vi "Sample Array - Fix Ascii.vi"(11 "Sample Array In":string[](array[string])) -> (3 "Sample Array Out":string[](array[string]))   [LabVIEW 2012]
uses:
  Globals Wilt.vi
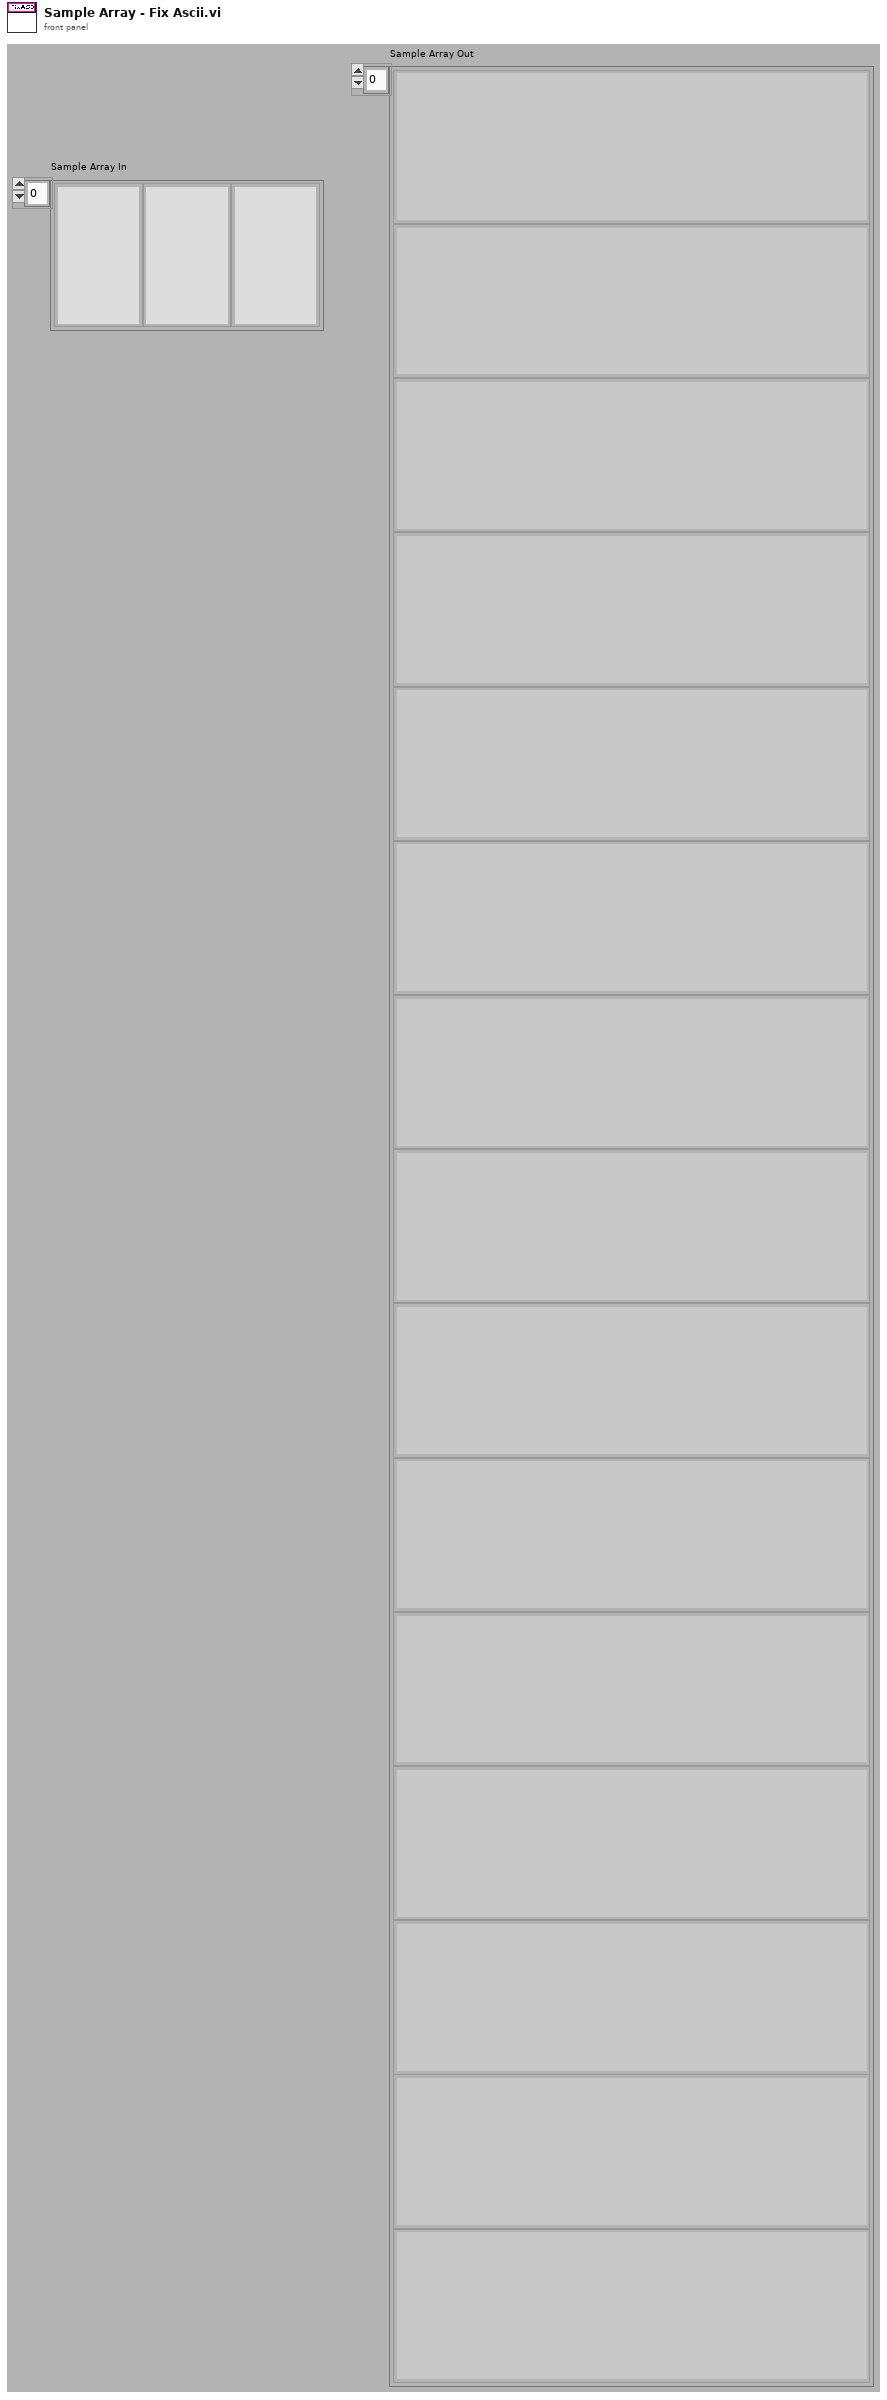
[diagram p1: front panel]
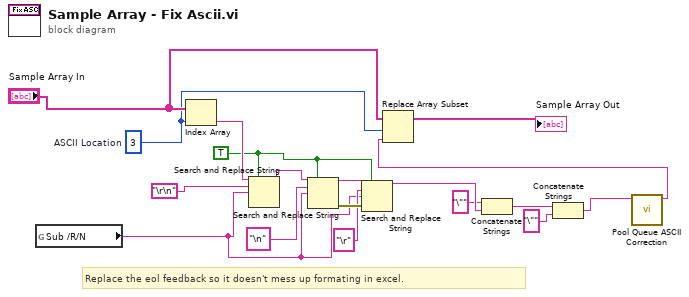
[diagram p0: block diagram]
diagram:
  w7 = TRUE ("replace all? (F)")
  w15 = 3  # ASCII Location
  # "Replace the eol feedback so it doesn't mess up formating in excel."
  n1 = global read "Globals Wilt.vi" "Sub /R/N"() -> (w8:string)
  n2 = Index Array(array="Sample Array In", index=w15) -> (element=w18:string)
  n3 = Search and Replace String(replace all?=w7, input string=w18, search string="\r\n", replace string=w8) -> (result string=w13:string)  [unwired: 4 in, 3 out]
  n4 = Search and Replace String(replace all?=w7, input string=w13, search string="\n", replace string=w8) -> (result string=w11:string, error out=w10:errorcluster)  [unwired: 4 in, 2 out]
  n5 = Search and Replace String(replace all?=w7, input string=w11, search string="\r", replace string=w8, error in=w10) -> (result string=w6:string)  [unwired: 3 in, 3 out]
  n6 = Concatenate Strings("\"" ("string"), w6) -> (w4:string)
  n7 = Concatenate Strings(w4, "\"" ("string")) -> (w2:string)
  n8 = call "Pool Queue ASCII Correction.vi"("Uncorrected Data"=w2) -> ("Corrected Data"=w1:string)  [unwired: 10 in]
  n9 = Replace Array Subset(array="Sample Array In", new element=w1, index=w15) -> (→"Sample Array Out":string[])
